vi "Test Case, String Compare.vi"() -> ()   [LabVIEW 2010]
panel:
  out "x = y?":bool
  in  "s2":string="ProgramNumber=2\\r ProgramDefined=YES\\r ProgramDisabled=NO\\r ProgramName=Program 2\\r ProgramFreqTable[00]Allowed=YES\\r ProgramFreqTable[01]Allowed=YES\\r ProgramFreqTable[02]Allowed=YES\\r ProgramFreqTable[03]Allowed=YES\\r ProgramFreqTable[04]Allowed=YES\\r ProgramFreqTable[05]Allowed=YES\\r ProgramFreqTable[06]Allowed=YES\\r ProgramFreqTable[07]Allowed=YES\\r ProgramFreqTable[08]Allowed=YES\\r ProgramFreqTable[09]Allowed=YES\\r ProgramFreqTable[10]Allowed=YES\\r ProgramFreqTable[11]Allowed=YES\\r ProgramFreqTable[12]Allowed=YES\\r ProgramFreqTable[13]Allowed=YES\\r ProgramFreqTable[14]Allowed=YES\\r ProgramFreqTable[15]Allowed=YES\\r ProgramFreqTable[16]Allowed=YES\\r ProgramFreqTable[17]Allowed=YES\\r ProgramFreqTable[18]Allowed=YES\\r ProgramFreqTable[19]Allowed=YES\\r ProgramFreqTable[20]Allowed=YES\\r ProgramFreqTable[21]Allowed=YES\\r ProgramFreqTable[22]Allowed=YES\\r ProgramFreqTable[23]Allowed=YES\\r ProgramFreqTable[24]Allowed=YES\\r ProgramFreqTable[25]Allowed=YES\\r ProgramFreqTable[26]Allowed=YES\\r ProgramFreqTable[27]Allowed=YES\\r ProgramFreqTable[28]Allowed=YES\\r ProgramFreqTable[29]Allowed=YES\\r ProgramFreqTable[30]Allowed=YES\\r ProgramFreqTable[31]Allowed=YES\\r ProgramFreqTable[32]Allowed=YES\\r ProgramFreqTable[33]Allowed=YES\\r ProgramFreqTable[34]Allowed=YES\\r ProgramFreqTable[35]Allowed=YES\\r ProgramFreqTable[36]Allowed=YES\\r ProgramFreqTable[37]Allowed=YES\\r ProgramFreqTable[38]Allowed=YES\\r ProgramFreqTable[39]Allowed=YES\\r ProgramFreqTable[40]Allowed=YES\\r ProgramFreqTable[41]Allowed=YES\\r ProgramFreqTable[42]Allowed=YES\\r ProgramFreqTable[43]Allowed=YES\\r ProgramFreqTable[44]Allowed=YES\\r ProgramFreqTable[45]Allowed=YES\\r ProgramFreqTable[46]Allowed=YES\\r ProgramFreqTable[47]Allowed=YES\\r ProgramFreqTable[48]Allowed=YES\\r ProgramFreqTable[49]Allowed=YES\\r ProgramFreqTable[50]Allowed=YES\\r ProgramFreqTable[51]Allowed=YES\\r ProgramFreqTable[52]Allowed=YES\\r ProgramFreqTable[53]Allowed=YES\\r ProgramFreqTable[54]Allowed=YES\\r ProgramFreqTable[55]Allowed=YES\\r ProgramFreqTable[56]Allowed=YES\\r ProgramFreqTable[57]Allowed=YES\\r ProgramFreqTable[58]Allowed=YES\\r ProgramFreqTable[59]Allowed=YES\\r ProgramFreqTable[60]Allowed=YES\\r ProgramFreqTable[61]Allowed=YES\\r ProgramFreqTable[62]Allowed=YES\\r ProgramFreqTable[63]Allowed=YES\\r ProgramFrequencyIndex=0\\r PA_Defined=YES\\r PB_Defined=YES\\r PC_Defined=YES\\r PD_Defined=YES\\r \\r -- PULSE PA --\\r PulseNamePA=P1\\r AmplitudeLowLimitPA=15\\r AmplitudeStepPA=15\\r AmplitudeStepIndexPA=1\\r PulseWidthLowLimitPA=10\\r PulseWidthHighLimitPA=20\\r PulseWidthPA=10\\r ElectrodeAmpPercentPA[CH01]=0\\r ElectrodeAmpPercentPA[CH02]=0\\r ElectrodeAmpPercentPA[CH03]=0\\r ElectrodeAmpPercentPA[CH04]=0\\r ElectrodeAmpPercentPA[CH05]=0\\r ElectrodeAmpPercentPA[CH06]=0\\r ElectrodeAmpPercentPA[CH07]=0\\r ElectrodeAmpPercentPA[CH08]=0\\r ElectrodeAmpPercentPA[CH09]=0\\r ElectrodeAmpPercentPA[CH10]=0\\r ElectrodeAmpPercentPA[CH11]=0\\r ElectrodeAmpPercentPA[CH12]=0\\r ElectrodeAmpPercentPA[CH13]=0\\r ElectrodeAmpPercentPA[CH14]=0\\r ElectrodeAmpPercentPA[CH15]=0\\r ElectrodeAmpPercentPA[CH16]=0\\r ElectrodeAmpPercentPA[CH17]=0\\r ElectrodeAmpPercentPA[CH18]=0\\r ElectrodeAmpPercentPA[CH19]=0\\r ElectrodeAmpPercentPA[CH20]=0\\r ElectrodeAmpPercentPA[CH21]=0\\r ElectrodeAmpPercentPA[CH22]=0\\r ElectrodeAmpPercentPA[CH23]=0\\r ElectrodeAmpPercentPA[CH24]=0\\r ElectrodeAmpPercentPA[CH25]=-100\\r ElectrodeAmpPercentPA[CH26]=100\\r \\r -- PULSE PB --\\r PulseNamePB=P2\\r AmplitudeLowLimitPB=15\\r AmplitudeStepPB=15\\r AmplitudeStepIndexPB=1\\r PulseWidthLowLimitPB=10\\r PulseWidthHighLimitPB=20\\r PulseWidthPB=10\\r ElectrodeAmpPercentPB[CH01]=0\\r ElectrodeAmpPercentPB[CH02]=0\\r ElectrodeAmpPercentPB[CH03]=0\\r ElectrodeAmpPercentPB[CH04]=0\\r ElectrodeAmpPercentPB[CH05]=0\\r ElectrodeAmpPercentPB[CH06]=0\\r ElectrodeAmpPercentPB[CH07]=0\\r ElectrodeAmpPercentPB[CH08]=0\\r ElectrodeAmpPercentPB[CH09]=0\\r ElectrodeAmpPercentPB[CH10]=0\\r ElectrodeAmpPercentPB[CH11]=0\\r ElectrodeAmpPercentPB[CH12]=0\\r ElectrodeAmpPercentPB[CH13]=0\\r ElectrodeAmpPercentPB[CH14]=0\\r ElectrodeAmpPercentPB[CH15]=0\\r ElectrodeAmpPercentPB[CH16]=0\\r ElectrodeAmpPercentPB[CH17]=0\\r ElectrodeAmpPercentPB[CH18]=0\\r ElectrodeAmpPercentPB[CH19]=0\\r ElectrodeAmpPercentPB[CH20]=0\\r ElectrodeAmpPercentPB[CH21]=0\\r ElectrodeAmpPercentPB[CH22]=0\\r ElectrodeAmpPercentPB[CH23]=0\\r ElectrodeAmpPercentPB[CH24]=0\\r ElectrodeAmpPercentPB[CH25]=-100\\r ElectrodeAmpPercentPB[CH26]=100\\r \\r -- PULSE PC --\\r PulseNamePC=P3\\r AmplitudeLowLimitPC=15\\r AmplitudeStepPC=15\\r AmplitudeStepIndexPC=1\\r PulseWidthLowLimitPC=10\\r PulseWidthHighLimitPC=20\\r PulseWidthPC=10\\r ElectrodeAmpPercentPC[CH01]=0\\r ElectrodeAmpPercentPC[CH02]=0\\r ElectrodeAmpPercentPC[CH03]=0\\r ElectrodeAmpPercentPC[CH04]=0\\r ElectrodeAmpPercentPC[CH05]=0\\r ElectrodeAmpPercentPC[CH06]=0\\r ElectrodeAmpPercentPC[CH07]=0\\r ElectrodeAmpPercentPC[CH08]=0\\r ElectrodeAmpPercentPC[CH09]=0\\r ElectrodeAmpPercentPC[CH10]=0\\r ElectrodeAmpPercentPC[CH11]=0\\r ElectrodeAmpPercentPC[CH12]=0\\r ElectrodeAmpPercentPC[CH13]=0\\r ElectrodeAmpPercentPC[CH14]=0\\r ElectrodeAmpPercentPC[CH15]=0\\r ElectrodeAmpPercentPC[CH16]=0\\r ElectrodeAmpPercentPC[CH17]=0\\r ElectrodeAmpPercentPC[CH18]=0\\r ElectrodeAmpPercentPC[CH19]=0\\r ElectrodeAmpPercentPC[CH20]=0\\r ElectrodeAmpPercentPC[CH21]=0\\r ElectrodeAmpPercentPC[CH22]=0\\r ElectrodeAmpPercentPC[CH23]=0\\r ElectrodeAmpPercentPC[CH24]=0\\r ElectrodeAmpPercentPC[CH25]=-100\\r ElectrodeAmpPercentPC[CH26]=100\\r \\r -- PULSE PD --\\r PulseNamePD=P4\\r AmplitudeLowLimitPD=15\\r AmplitudeStepPD=15\\r AmplitudeStepIndexPD=1\\r PulseWidthLowLimitPD=10\\r PulseWidthHighLimitPD=20\\r PulseWidthPD=10\\r ElectrodeAmpPercentPD[CH01]=0\\r ElectrodeAmpPercentPD[CH02]=0\\r ElectrodeAmpPercentPD[CH03]=0\\r ElectrodeAmpPercentPD[CH04]=0\\r ElectrodeAmpPercentPD[CH05]=0\\r ElectrodeAmpPercentPD[CH06]=0\\r ElectrodeAmpPercentPD[CH07]=0\\r ElectrodeAmpPercentPD[CH08]=0\\r ElectrodeAmpPercentPD[CH09]=0\\r ElectrodeAmpPercentPD[CH10]=0\\r ElectrodeAmpPercentPD[CH11]=0\\r ElectrodeAmpPercentPD[CH12]=0\\r ElectrodeAmpPercentPD[CH13]=0\\r ElectrodeAmpPercentPD[CH14]=0\\r ElectrodeAmpPercentPD[CH15]=0\\r ElectrodeAmpPercentPD[CH16]=0\\r ElectrodeAmpPercentPD[CH17]=0\\r ElectrodeAmpPercentPD[CH18]=0\\r ElectrodeAmpPercentPD[CH19]=0\\r ElectrodeAmpPercentPD[CH20]=0\\r ElectrodeAmpPercentPD[CH21]=0\\r ElectrodeAmpPercentPD[CH22]=0\\r ElectrodeAmpPercentPD[CH23]=0\\r ElectrodeAmpPercentPD[CH24]=0\\r ElectrodeAmpPercentPD[CH25]=-100\\r ElectrodeAmpPercentPD[CH26]=100"
  in  "s1":string="ProgramNumber=1\\r ProgramDefined=YES\\r ProgramDisabled=NO\\r ProgramName=Program 1\\r ProgramFreqTable[00]Allowed=YES\\r ProgramFreqTable[01]Allowed=YES\\r ProgramFreqTable[02]Allowed=YES\\r ProgramFreqTable[03]Allowed=YES\\r ProgramFreqTable[04]Allowed=YES\\r ProgramFreqTable[05]Allowed=YES\\r ProgramFreqTable[06]Allowed=YES\\r ProgramFreqTable[07]Allowed=YES\\r ProgramFreqTable[08]Allowed=YES\\r ProgramFreqTable[09]Allowed=YES\\r ProgramFreqTable[10]Allowed=YES\\r ProgramFreqTable[11]Allowed=YES\\r ProgramFreqTable[12]Allowed=YES\\r ProgramFreqTable[13]Allowed=YES\\r ProgramFreqTable[14]Allowed=YES\\r ProgramFreqTable[15]Allowed=YES\\r ProgramFreqTable[16]Allowed=YES\\r ProgramFreqTable[17]Allowed=YES\\r ProgramFreqTable[18]Allowed=YES\\r ProgramFreqTable[19]Allowed=YES\\r ProgramFreqTable[20]Allowed=YES\\r ProgramFreqTable[21]Allowed=YES\\r ProgramFreqTable[22]Allowed=YES\\r ProgramFreqTable[23]Allowed=YES\\r ProgramFreqTable[24]Allowed=YES\\r ProgramFreqTable[25]Allowed=YES\\r ProgramFreqTable[26]Allowed=YES\\r ProgramFreqTable[27]Allowed=YES\\r ProgramFreqTable[28]Allowed=YES\\r ProgramFreqTable[29]Allowed=YES\\r ProgramFreqTable[30]Allowed=YES\\r ProgramFreqTable[31]Allowed=YES\\r ProgramFreqTable[32]Allowed=YES\\r ProgramFreqTable[33]Allowed=YES\\r ProgramFreqTable[34]Allowed=YES\\r ProgramFreqTable[35]Allowed=YES\\r ProgramFreqTable[36]Allowed=YES\\r ProgramFreqTable[37]Allowed=YES\\r ProgramFreqTable[38]Allowed=YES\\r ProgramFreqTable[39]Allowed=YES\\r ProgramFreqTable[40]Allowed=YES\\r ProgramFreqTable[41]Allowed=YES\\r ProgramFreqTable[42]Allowed=YES\\r ProgramFreqTable[43]Allowed=YES\\r ProgramFreqTable[44]Allowed=YES\\r ProgramFreqTable[45]Allowed=YES\\r ProgramFreqTable[46]Allowed=YES\\r ProgramFreqTable[47]Allowed=YES\\r ProgramFreqTable[48]Allowed=YES\\r ProgramFreqTable[49]Allowed=YES\\r ProgramFreqTable[50]Allowed=YES\\r ProgramFreqTable[51]Allowed=YES\\r ProgramFreqTable[52]Allowed=YES\\r ProgramFreqTable[53]Allowed=YES\\r ProgramFreqTable[54]Allowed=YES\\r ProgramFreqTable[55]Allowed=YES\\r ProgramFreqTable[56]Allowed=YES\\r ProgramFreqTable[57]Allowed=YES\\r ProgramFreqTable[58]Allowed=YES\\r ProgramFreqTable[59]Allowed=YES\\r ProgramFreqTable[60]Allowed=YES\\r ProgramFreqTable[61]Allowed=YES\\r ProgramFreqTable[62]Allowed=YES\\r ProgramFreqTable[63]Allowed=YES\\r ProgramFrequencyIndex=0\\r PA_Defined=YES\\r PB_Defined=YES\\r PC_Defined=YES\\r PD_Defined=YES\\r \\r -- PULSE PA --\\r PulseNamePA=P1\\r AmplitudeLowLimitPA=15\\r AmplitudeStepPA=15\\r AmplitudeStepIndexPA=1\\r PulseWidthLowLimitPA=10\\r PulseWidthHighLimitPA=20\\r PulseWidthPA=10\\r ElectrodeAmpPercentPA[CH01]=0\\r ElectrodeAmpPercentPA[CH02]=0\\r ElectrodeAmpPercentPA[CH03]=0\\r ElectrodeAmpPercentPA[CH04]=0\\r ElectrodeAmpPercentPA[CH05]=0\\r ElectrodeAmpPercentPA[CH06]=0\\r ElectrodeAmpPercentPA[CH07]=0\\r ElectrodeAmpPercentPA[CH08]=0\\r ElectrodeAmpPercentPA[CH09]=0\\r ElectrodeAmpPercentPA[CH10]=0\\r ElectrodeAmpPercentPA[CH11]=0\\r ElectrodeAmpPercentPA[CH12]=0\\r ElectrodeAmpPercentPA[CH13]=0\\r ElectrodeAmpPercentPA[CH14]=0\\r ElectrodeAmpPercentPA[CH15]=0\\r ElectrodeAmpPercentPA[CH16]=0\\r ElectrodeAmpPercentPA[CH17]=0\\r ElectrodeAmpPercentPA[CH18]=0\\r ElectrodeAmpPercentPA[CH19]=0\\r ElectrodeAmpPercentPA[CH20]=0\\r ElectrodeAmpPercentPA[CH21]=0\\r ElectrodeAmpPercentPA[CH22]=0\\r ElectrodeAmpPercentPA[CH23]=0\\r ElectrodeAmpPercentPA[CH24]=0\\r ElectrodeAmpPercentPA[CH25]=-100\\r ElectrodeAmpPercentPA[CH26]=100\\r \\r -- PULSE PB --\\r PulseNamePB=P2\\r AmplitudeLowLimitPB=15\\r AmplitudeStepPB=15\\r AmplitudeStepIndexPB=1\\r PulseWidthLowLimitPB=10\\r PulseWidthHighLimitPB=20\\r PulseWidthPB=10\\r ElectrodeAmpPercentPB[CH01]=0\\r ElectrodeAmpPercentPB[CH02]=0\\r ElectrodeAmpPercentPB[CH03]=0\\r ElectrodeAmpPercentPB[CH04]=0\\r ElectrodeAmpPercentPB[CH05]=0\\r ElectrodeAmpPercentPB[CH06]=0\\r ElectrodeAmpPercentPB[CH07]=0\\r ElectrodeAmpPercentPB[CH08]=0\\r ElectrodeAmpPercentPB[CH09]=0\\r ElectrodeAmpPercentPB[CH10]=0\\r ElectrodeAmpPercentPB[CH11]=0\\r ElectrodeAmpPercentPB[CH12]=0\\r ElectrodeAmpPercentPB[CH13]=0\\r ElectrodeAmpPercentPB[CH14]=0\\r ElectrodeAmpPercentPB[CH15]=0\\r ElectrodeAmpPercentPB[CH16]=0\\r ElectrodeAmpPercentPB[CH17]=0\\r ElectrodeAmpPercentPB[CH18]=0\\r ElectrodeAmpPercentPB[CH19]=0\\r ElectrodeAmpPercentPB[CH20]=0\\r ElectrodeAmpPercentPB[CH21]=0\\r ElectrodeAmpPercentPB[CH22]=0\\r ElectrodeAmpPercentPB[CH23]=0\\r ElectrodeAmpPercentPB[CH24]=0\\r ElectrodeAmpPercentPB[CH25]=-100\\r ElectrodeAmpPercentPB[CH26]=100\\r \\r -- PULSE PC --\\r PulseNamePC=P3\\r AmplitudeLowLimitPC=15\\r AmplitudeStepPC=15\\r AmplitudeStepIndexPC=1\\r PulseWidthLowLimitPC=10\\r PulseWidthHighLimitPC=20\\r PulseWidthPC=10\\r ElectrodeAmpPercentPC[CH01]=0\\r ElectrodeAmpPercentPC[CH02]=0\\r ElectrodeAmpPercentPC[CH03]=0\\r ElectrodeAmpPercentPC[CH04]=0\\r ElectrodeAmpPercentPC[CH05]=0\\r ElectrodeAmpPercentPC[CH06]=0\\r ElectrodeAmpPercentPC[CH07]=0\\r ElectrodeAmpPercentPC[CH08]=0\\r ElectrodeAmpPercentPC[CH09]=0\\r ElectrodeAmpPercentPC[CH10]=0\\r ElectrodeAmpPercentPC[CH11]=0\\r ElectrodeAmpPercentPC[CH12]=0\\r ElectrodeAmpPercentPC[CH13]=0\\r ElectrodeAmpPercentPC[CH14]=0\\r ElectrodeAmpPercentPC[CH15]=0\\r ElectrodeAmpPercentPC[CH16]=0\\r ElectrodeAmpPercentPC[CH17]=0\\r ElectrodeAmpPercentPC[CH18]=0\\r ElectrodeAmpPercentPC[CH19]=0\\r ElectrodeAmpPercentPC[CH20]=0\\r ElectrodeAmpPercentPC[CH21]=0\\r ElectrodeAmpPercentPC[CH22]=0\\r ElectrodeAmpPercentPC[CH23]=0\\r ElectrodeAmpPercentPC[CH24]=0\\r ElectrodeAmpPercentPC[CH25]=-100\\r ElectrodeAmpPercentPC[CH26]=100\\r \\r -- PULSE PD --\\r PulseNamePD=P4\\r AmplitudeLowLimitPD=15\\r AmplitudeStepPD=15\\r AmplitudeStepIndexPD=1\\r PulseWidthLowLimitPD=10\\r PulseWidthHighLimitPD=20\\r PulseWidthPD=10\\r ElectrodeAmpPercentPD[CH01]=0\\r ElectrodeAmpPercentPD[CH02]=0\\r ElectrodeAmpPercentPD[CH03]=0\\r ElectrodeAmpPercentPD[CH04]=0\\r ElectrodeAmpPercentPD[CH05]=0\\r ElectrodeAmpPercentPD[CH06]=0\\r ElectrodeAmpPercentPD[CH07]=0\\r ElectrodeAmpPercentPD[CH08]=0\\r ElectrodeAmpPercentPD[CH09]=0\\r ElectrodeAmpPercentPD[CH10]=0\\r ElectrodeAmpPercentPD[CH11]=0\\r ElectrodeAmpPercentPD[CH12]=0\\r ElectrodeAmpPercentPD[CH13]=0\\r ElectrodeAmpPercentPD[CH14]=0\\r ElectrodeAmpPercentPD[CH15]=0\\r ElectrodeAmpPercentPD[CH16]=0\\r ElectrodeAmpPercentPD[CH17]=0\\r ElectrodeAmpPercentPD[CH18]=0\\r ElectrodeAmpPercentPD[CH19]=0\\r ElectrodeAmpPercentPD[CH20]=0\\r ElectrodeAmpPercentPD[CH21]=0\\r ElectrodeAmpPercentPD[CH22]=0\\r ElectrodeAmpPercentPD[CH23]=0\\r ElectrodeAmpPercentPD[CH24]=0\\r ElectrodeAmpPercentPD[CH25]=-100\\r ElectrodeAmpPercentPD[CH26]=100"
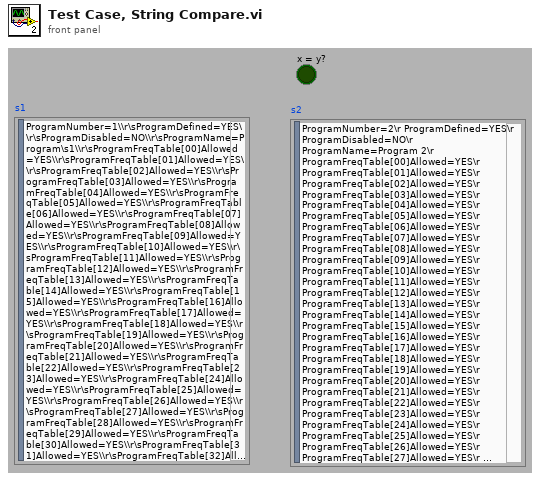
[diagram p1: front panel]
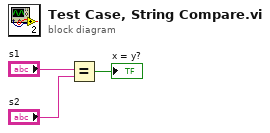
[diagram p0: block diagram]
diagram:
  n1 = Equal?(x="s1", y="s2") -> (x = y?=→"x = y?":bool)
